vi "02 - Programming Structures.vi"   [LabVIEW 2025]
panel:
  # "Open Block Diagram to Browse Syntax\nCtl + E (instructions on diagram)"
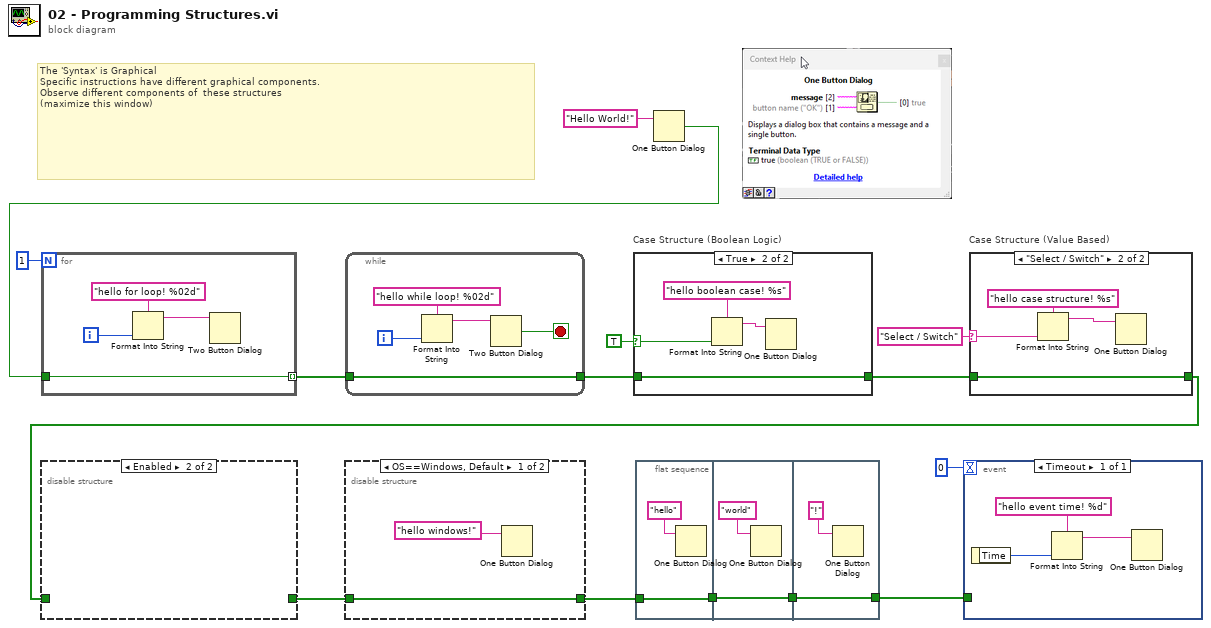
[diagram p0: block diagram]
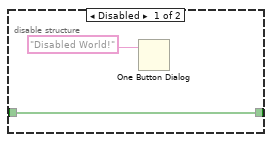
[diagram p3: hidden frame]
diagram:
  # "The 'Syntax' is Graphical\nSpecific instructions have different graphical components.\nObserve different components of  these structures\n(maximize this window)"
  n1 = flat-sequence {
    tunnel: [w16] -> w10
    tunnel: w9 -> [w16]
    tunnel: [w18] -> w11
    tunnel: w10 -> [w18]
    tunnel: [w20] -> w12
    tunnel: w11 -> [w20]
    frame #0 {
      n2 = One Button Dialog(message="hello") -> ()  [unwired: 1 in, 1 out]
    }
    frame #1 {
      n3 = One Button Dialog(message="world") -> ()  [unwired: 1 in, 1 out]
    }
    frame #2 {
      n4 = One Button Dialog(message="!") -> ()  [unwired: 1 in, 1 out]
    }
  }
  n5 = One Button Dialog(message="Hello World!") -> (true=w1:bool)  [unwired: 1 in]
  n6 = for {
    N: 1 -> [_]
    tunnel: [w22] -> w5 mode=indexing
    tunnel: w1 -> [w22]
    i -> [w25]
    n7 = Format Into String(format string="hello for loop! %02d", w25) -> (resulting string=w24:string)  [unwired: 2 in, 1 out]
    n8 = Two Button Dialog(message=w24) -> ()  [unwired: 2 in, 1 out]
  }
  n9 = while {
    tunnel: [w26] -> w6
    tunnel: w5 -> [w26]
    i -> [w28]
    stop <- w27 stop-if-true
    n10 = Format Into String(format string="hello while loop! %02d", w28) -> (resulting string=w29:string)  [unwired: 2 in, 1 out]
    n11 = Two Button Dialog(message=w29) -> (T button?=w27:bool)  [unwired: 2 in]
  }
  n12 = case "Case Structure (Boolean Logic)" shown="True" TRUE {
    selector: TRUE -> [_ w34]
    tunnel: [_ w31] -> w7
    tunnel: w6 -> [_ w31]
    frame False {
    }
    frame True {
      n13 = Format Into String(format string="hello boolean case! %s", w34) -> (resulting string=w33:string)  [unwired: 2 in, 1 out]
      n14 = One Button Dialog(message=w33) -> ()  [unwired: 1 in, 1 out]
    }
  }
  n15 = event shown="[0] Timeout" {
    selector: _ -> [_]
    dyn-events: _ -> [_]
    timeout: 0 -> [_]
    tunnel: w12 -> [_]
    event Timeout {
      n16 = event-data() -> ("Time"=w37:u32)  [unwired: 1 in]
      n17 = Format Into String(format string="hello event time! %d" ("message"), w37) -> (resulting string=w35:string)  [unwired: 2 in, 1 out]
      n18 = One Button Dialog(message=w35) -> ()  [unwired: 1 in, 1 out]
    }
  }
  n19 = case "Case Structure (Value Based)" shown="\"Select / Switch\"" "Select / Switch" {
    selector: "Select / Switch" -> [_ w41]
    tunnel: [w38 w39] -> w3
    tunnel: w7 -> [w38 w39]
    frame Default {
    }
    frame "Select / Switch" {
      n20 = Format Into String(format string="hello case structure! %s", w41) -> (resulting string=w40:string)  [unwired: 2 in, 1 out]
      n21 = One Button Dialog(message=w40) -> ()  [unwired: 1 in, 1 out]
    }
  }
  n22 = disable-structure "Diagram Disable Structure" shown="Enabled" {
    disable-tunnel: [w43 _] -> w8
    disable-tunnel: w3 -> [w43 _]
    frame Disabled {
      n23 = One Button Dialog(message="Disabled World!") -> ()  [unwired: 1 in, 1 out]
    }
    frame Enabled {
    }
  }
  n24 = disable-structure "Conditional Disable Structure" shown="OS==Windows, Default" {
    disable-tunnel: [w45 _] -> w9
    disable-tunnel: w8 -> [w45 _]
    frame condition #0 (active) {
      n25 = One Button Dialog(message="hello windows!") -> ()  [unwired: 1 in, 1 out]
    }
    frame condition #1 {
    }
  }
